vi "GenerateUniqueFilename.vi"(7 "format string":string="%03d", 8 "error in (no error)":errorcluster, 9 "File Name Suffixes":string[](array[string]), 10 "File Name Prefix":string, 11 "Folder":string="c:\\data\\") -> (0 "error out":errorcluster, 3 "Paths":path[](array[path]))   [LabVIEW 2021]
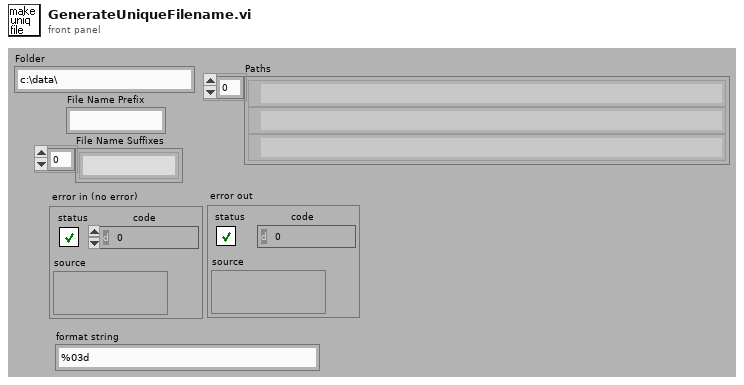
[diagram p1: front panel]
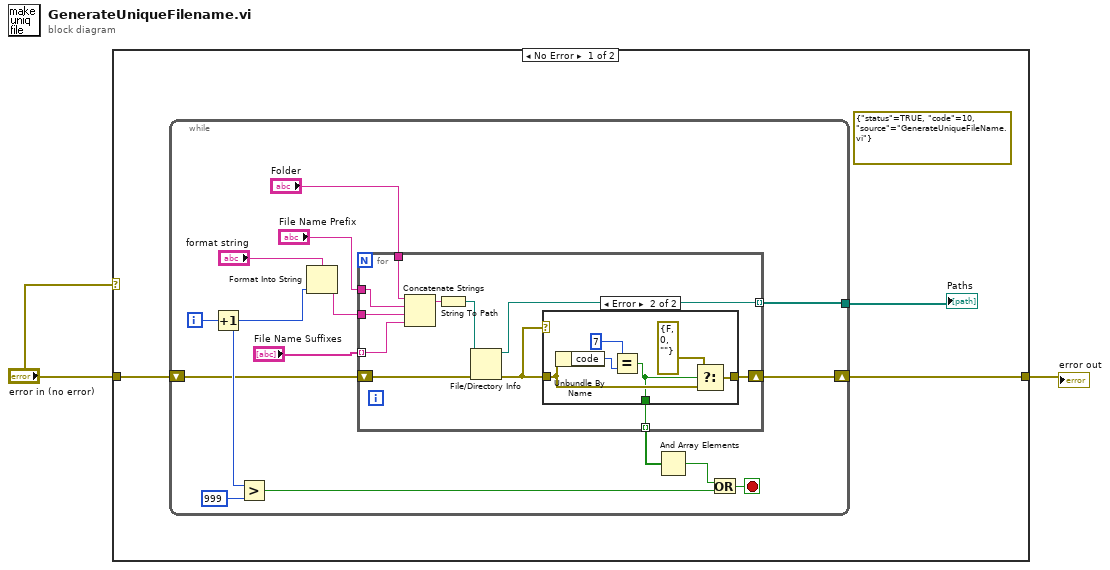
[diagram p0: block diagram]
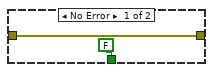
[diagram p2: hidden frame]
diagram:
  n1 = case shown="No Error" "error in (no error)" {
    tunnel: "error in (no error)" -> [w4 w40]
    tunnel: [w3 w40] -> w2
    frame No Error {
      (unwired) errorcluster {"status"=TRUE, "code"=10, "source"="GenerateUniqueFileName.vi"} ("f")
      n2 = while {
        tunnel: [w15] -> w5
        shift-right: [w11] -> w3
        shift-left: w4 -> [w10]
        i -> [w20]
        stop <- w16 stop-if-true
        n3 = Increment(x=w20) -> (x+1=w18:i32)
        n4 = Greater?(x=w18, y=999) -> (0:w14:bool)
        n5 = Format Into String(format string="format string", w18) -> (resulting string=w19:string)  [unwired: 2 in, 1 out]
        n6 = for {
          tunnel: w19 -> [w31]
          tunnel: [w28] -> w15 mode=indexing
          tunnel: "Folder" -> [w27]
          tunnel: "File Name Suffixes" -> [w26] mode=indexing
          shift-right: [w24] -> w11
          shift-left: w10 -> [w25]
          tunnel: [w22] -> w9 mode=indexing
          tunnel: "File Name Prefix" -> [w21]
          n7 = Concatenate Strings(w27, w21, w31, w26) -> (w29:string)
          n8 = String To Path(string=w29) -> (path=w30:path)
          n9 = File/Directory Info(path=w30, error in=w25) -> (path out=w28:path, error out=w23:errorcluster)  [unwired: 5 out]
          n10 = case shown="Error" w23 {
            tunnel: [w33 w39] -> w24
            tunnel: w23 -> [w33 w36]
            tunnel: [FALSE w34] -> w22
            frame No Error {
            }
            frame Error {
              n11 = Unbundle By Name(w36) -> ("code"=w38:i32)
              n12 = Equal?(x=7 ("y"), y=w38) -> (x = y?=w34:bool)
              n13 = Select(t=errorcluster {"status"=FALSE, "code"=0, "source"=""}, s=w34, f=w36) -> (s? t:f=w39:errorcluster)
            }
          }
        }
        n14 = And Array Elements(Boolean array=w9) -> (logical AND=w8:bool)
        n15 = Or(x=w8, y=w14) -> (x .or. y?=w16:bool)
      }
      "Paths" <- w5
    }
    frame Error {
    }
  }
  "error out" <- w2
